vi "Async Stop and get video from CamServer.vi"(1 "Video name":string="test", 2 "Video directory path":path=path "C:/test") -> (0 "Error out":errorcluster)   [LabVIEW 2016]
doc: "Asynchronously ends recording video from the selected camera on the camera server (previously started with \"Async Start....\") and saves the video to the specified path with specified name."
uses:
  Globals/CamServer global.vi
panel:
  # "PN 21/08/15"
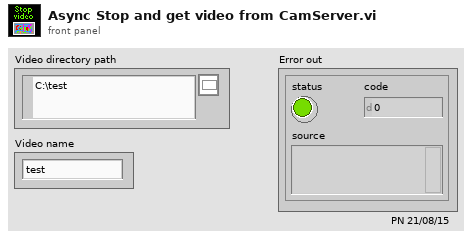
[diagram p1: front panel]
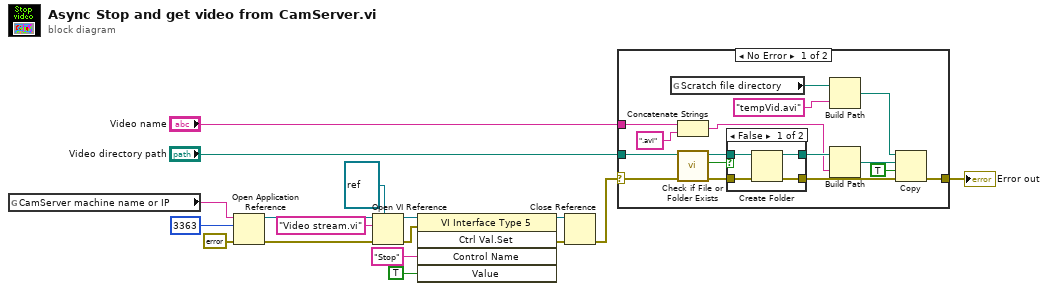
[diagram p0: block diagram]
diagram:
  n1 = global read "CamServer global.vi" "CamServer machine name or IP"() -> (w1:string)
  n2 = Open Application Reference(8:errorcluster {"status"=FALSE, "code"=0, "source"=""} ("error in (no error)"), 10:u16 3363 ("port"), 11:w1) -> (0:w11:errorcluster, 3:w12:refnum<vi>)  [unwired: 1 in]
  n3 = Open VI Reference(type specifier VI Refnum (for type only)=refnum<vi> refnum, application reference (local)=w12, vi path="Video stream.vi" ("machine name"), error in (no error)=w11) -> (vi reference=w8:refnum<vi>, error out=w5:errorcluster)  [unwired: 2 in]
  n4 = invoke class="VI Interface Type 5" method="Ctrl Val.Set"(reference=w8, error in=w5, "Control Name"="Stop", "Value"=TRUE) -> (reference out=w7:refnum<vi>, error out=w4:errorcluster)  [unwired: 1 in, 3 out]
  n5 = Close Reference(reference=w7, error in (no error)=w4) -> (error out=w3:errorcluster)
  n6 = case shown="No Error" w3 {
    selector: w3 -> [w32 w40]
    tunnel: "Video directory path" -> [w33 _]
    tunnel: "Video name" -> [w25 _]
    tunnel: [w23 w40] -> w15
    frame No Error {
      n7 = global read "CamServer global.vi" "Scratch file directory"() -> (w19:path)
      n8 = Concatenate Strings(w25, ".avi" ("string")) -> (w22:string)
      n9 = call <vilib>:"Check if File or Folder Exists.vi"("error in (no error)"=w32, "path"=w33) -> ("error out"=w29:errorcluster, "file or folder exists?"=w31:bool, "dup path"=w30:path)  [unwired: 7 in]
      n10 = case shown="False" w31 {
        tunnel: w30 -> [w37 w39]
        tunnel: w29 -> [w36 w38]
        tunnel: [w35 w39] -> w26
        tunnel: [w34 w38] -> w27
        frame False {
          n11 = Create Folder(path (use dialog)=w37, error in=w36) -> (created path=w35:path, error out=w34:errorcluster)  [unwired: 1 in, 1 out]
        }
        frame True {
        }
      }
      n12 = Build Path(base path=w19, name or relative path="tempVid.avi") -> (appended path=w18:path)
      n13 = Build Path(base path=w26, name or relative path=w22) -> (appended path=w24:path)
      n14 = Copy(8:w27, 9:TRUE ("overwrite (F)"), 10:w24, 11:w18) -> (0:w23:errorcluster)  [unwired: 1 in, 2 out]
    }
    frame Error {
    }
  }
  "Error out" <- w15
